vi "09T_input_temp_array.vi"(11 "List file adr":path) -> (2 "Temp_array":dbl[](array[numeric]), 3 "size":i32)   [LabVIEW 2017]
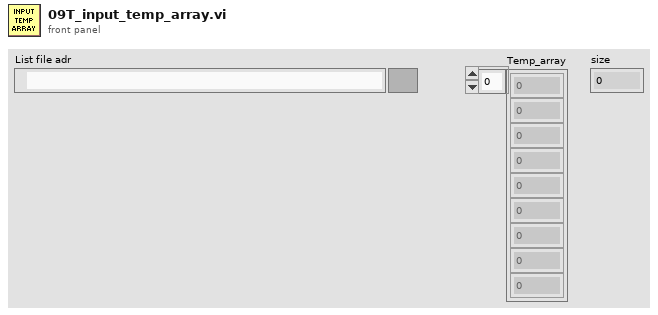
[diagram p1: front panel]
types:
  T1 = enum16{"open", "replace", "create", "open or create", "replace or create", "replace or create with confirmation"}
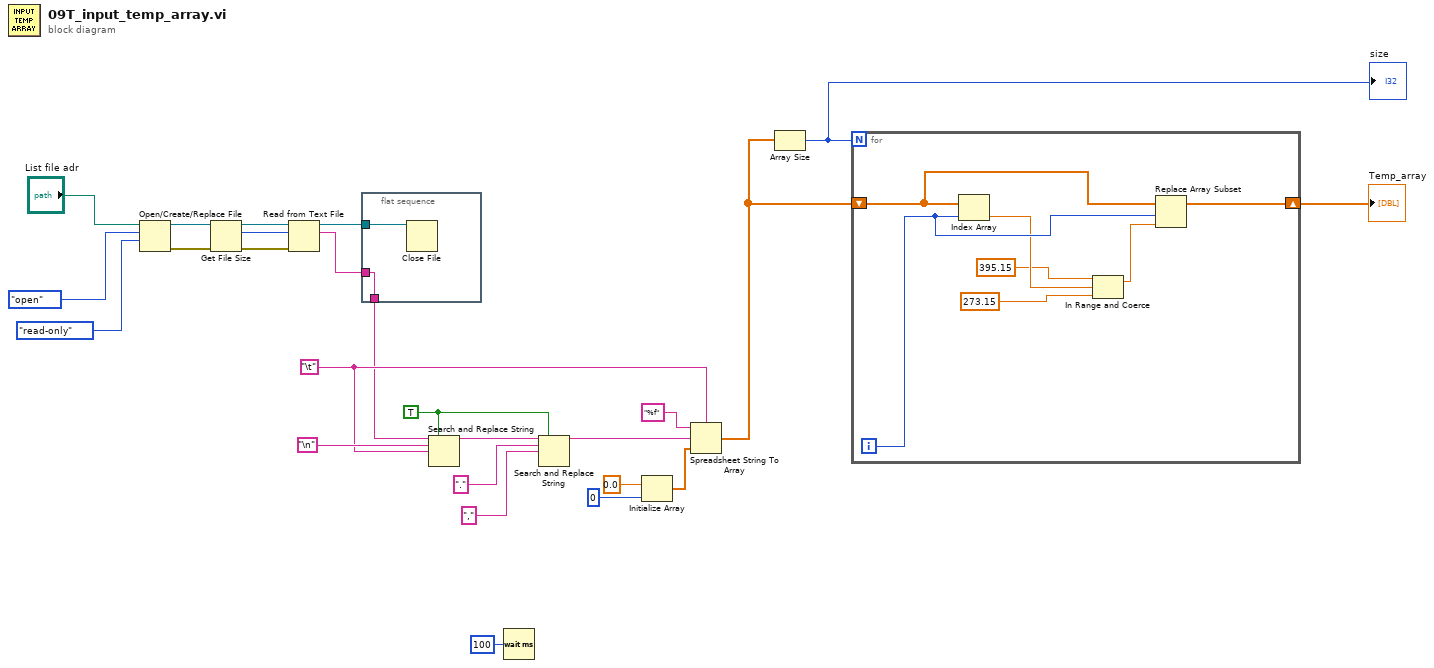
[diagram p0: block diagram]
diagram:
  w14 = "\t"
  w13 = TRUE ("replace all? (F)")
  n1 = Open/Create/Replace File(file path (use dialog)="List file adr", operation (0:open)=T1."open", access (0:read/write)=enum16{"read/write", "read-only", "write-only"}."read-only") -> (refnum out=w23:refnum<file>, error out=w22:errorcluster)  [unwired: 3 in, 1 out]
  n2 = Get File Size(file=w23, error in=w22) -> (refnum out=w19:refnum<file>, size (in bytes)=w20:i64, 0:w21:errorcluster)
  n3 = Read from Text File(file (use dialog)=w19, count=w20, error in=w21) -> (refnum out=w4:refnum<file>, text=w3:string)  [unwired: 1 in, 2 out]
  n4 = flat-sequence {
    tunnel: w4 -> [w28]
    tunnel: w3 -> [w27]
    tunnel: [w27] -> w2
    frame #0 {
      n5 = Close File(refnum=w28) -> ()  [unwired: 1 in, 2 out]
    }
  }
  n6 = Search and Replace String(replace all?=w13, input string=w2, search string="\n", replace string=w14) -> (result string=w8:string)  [unwired: 4 in, 3 out]
  n7 = Wait (ms)(milliseconds to wait=u32 100) -> ()  [unwired: 1 out]
  n8 = Search and Replace String(replace all?=w13, input string=w8, search string=".", replace string="," ("replace string (\"\")")) -> (result string=w10:string)  [unwired: 4 in, 3 out]
  n9 = Initialize Array(0.0, 0 ("dimension size")) -> (w16:dbl[])
  n10 = Spreadsheet String To Array(delimiter (Tab)=w14, format string="%f", spreadsheet string=w10, array type (2D Dbl)=w16) -> (array=w6:dbl[])
  n11 = Array Size(array=w6) -> (size(s)=w7:i32)
  "size" <- w7
  n12 = for {
    N: w7 -> [_]
    shift-right: [w29] -> w5
    shift-left: w6 -> [w30]
    i -> [w35]
    n13 = Index Array(array=w30, index=w35) -> (element=w34:dbl)
    n14 = In Range and Coerce(upper limit=395.15, x=w34, lower limit=273.15) -> (coerced(x)=w31:dbl)  [unwired: 1 out]
    n15 = Replace Array Subset(array=w30, new element=w31, index=w35) -> (w29:dbl[])
  }
  "Temp_array" <- w5
